vi "handle_connection.vi"(4 "WebSocket Logger":refnum<class "WebSocket Logger.lvclass">, 6 "hangup?":refnum<notifier>, 8 "error in (no error)":errorcluster, 10 "WebSocket Connection":refnum<class "WebSocket Connection.lvclass">, 11 "WebSocket Connection Handler in":refnum<class "WebSocket Connection Handler.lvclass">) -> (0 "error out":errorcluster)   [LabVIEW 2019, in "WebSocket Server Toolkit.lvlib" / "WebSocket Connection Handler.lvclass"]
doc: "<b>Description</b> WebSocket connection handler. Your implementation should continue running until a non-zero hangup notification is received.\n\n<b>Inputs</b>\n<b>WebSocket Logger</b>: A logger\n<b>WebSocket Connection</b>: The active connection. Read and Write to this connection.\n<b>hangup?</b>: An integer-typed notification that will fire if the client hangs up the connection."
uses:
  WebSocket Connection Handler.lvclass
  types/status_code.ctl
  WebSocket Connection/WebSocket Connection.lvclass
  WebSocket Server Toolkit.lvlib
  WebSocket Logger/WebSocket Logger.lvclass
panel:
  # "Handle messsages from the receive queue.\nSend messages on the send queue.\nReturn from the VI to hang-up the connection."
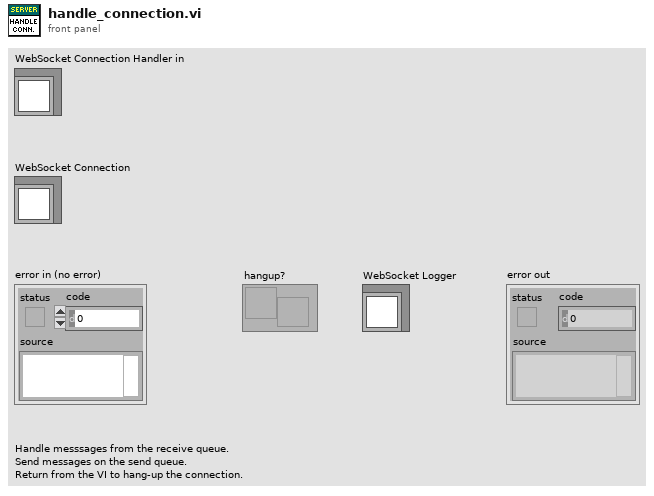
[diagram p1: front panel]
types:
  T1 = typedef "WebSocket Server Toolkit.lvlib/status_code.ctl" = u16
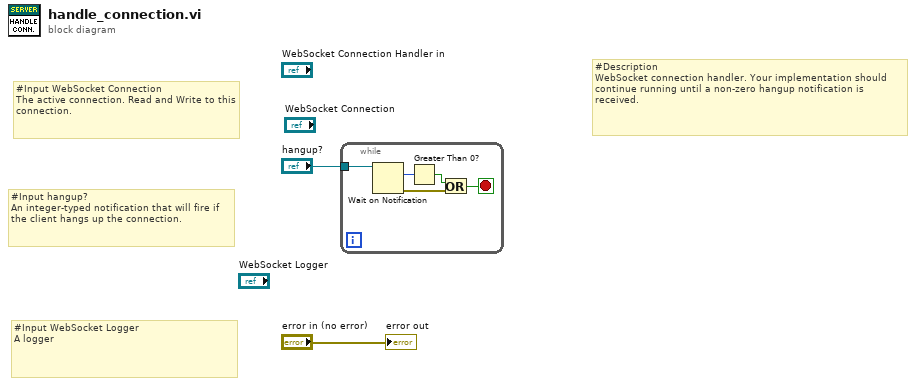
[diagram p0: block diagram]
diagram:
  # "#Input WebSocket Logger\nA logger"
  # "#Input WebSocket Connection\nThe active connection. Read and Write to this connection."
  # "#Input hangup?\nAn integer-typed notification that will fire if the client hangs up the connection."
  # "#Description\nWebSocket connection handler. Your implementation should continue running until a non-zero hangup notification is received."
  n1 = while {
    tunnel: "hangup?" -> [w7]
    stop <- w4 stop-if-true
    n2 = Wait on Notification(notifier=w7) -> (notification=w6:T1, error out=w5:errorcluster)  [unwired: 3 in, 2 out]
    n3 = Greater Than 0?(x=w6) -> (x > 0?=w3:bool)
    n4 = Or(x=w3, y=w5) -> (x .or. y?=w4:bool)
  }
  "error out" <- "error in (no error)"
